vi "Clear_Destinations.vi"(8 "error in (no error)":errorcluster, 11 "Installer in":refnum<class "Installer.lvclass">) -> (0 "error out":errorcluster, 3 "Installer out":refnum<class "Installer.lvclass">)   [LabVIEW 2020, in "Installer.lvclass"]
uses:
  <vilib>/AppBuilder/IB_Classes/Installer/Installer.lvclass
  <vilib>/AppBuilder/IB_Classes/Installer/Installer.lvclass/Installer.ctl
  <vilib>/AppBuilder/IB_Classes/Destination/IB_Destination.lvclass
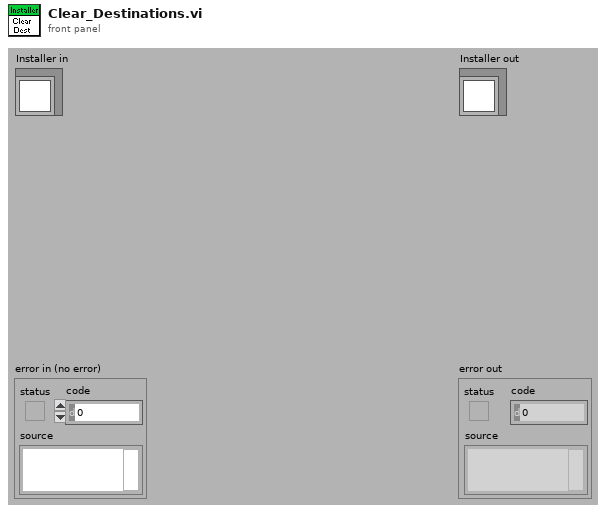
[diagram p1: front panel]
types:
  T1 = typedef "ItemRef.ctl" = u64
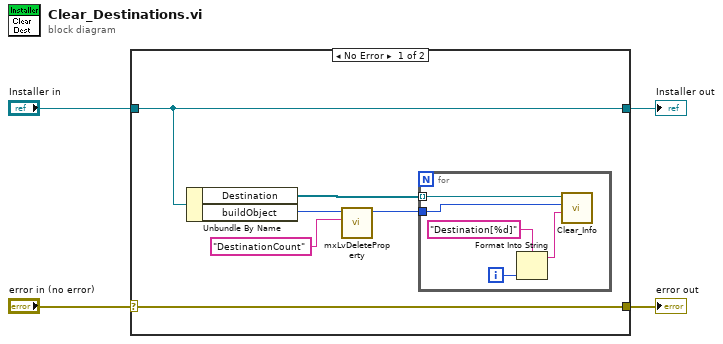
[diagram p0: block diagram]
diagram:
  n1 = case shown="No Error" "error in (no error)" {
    selector: "error in (no error)" -> [w10 w17]
    tunnel: [w10 w17] -> w3
    tunnel: [w8 w16] -> w1
    tunnel: "Installer in" -> [w8 w16]
    frame No Error {
      n2 = Unbundle By Name(w8) -> ("Destination"=w9:refnum<class "IB_Destination.lvclass">[], "buildObject"=w6:T1)
      n3 = call <resource>:"mxLvDeleteProperty.vi"("Tag"="DestinationCount", "Item"=w6) -> ("Item"=w5:T1)  [unwired: 1 in, 8 out]
      n4 = for {
        tunnel: w9 -> [w14] mode=indexing
        tunnel: w5 -> [w15]
        i -> [w11]
        n5 = Format Into String(format string="Destination[%d]", w11) -> (resulting string=w12:string)  [unwired: 2 in, 1 out]
        n6 = call <vilib>:"Clear_Info.vi"("index"=w12, "buildObject"=w15, "IB_Destination.lvclass"=w14) -> ()  [unwired: 7 in, 2 out]
      }
    }
    frame Error {
    }
  }
  "error out" <- w3
  "Installer out" <- w1
